vi "PrintDebugInfo.vi"(8 "error in (no error)":errorcluster, 11 "CLabVIEWContainer in":refnum<class "CLabVIEWContainer.lvclass">) -> (0 "error out":errorcluster, 1 "Debug string":string, 3 "CLabVIEWContainer out":refnum<class "CLabVIEWContainer.lvclass">)   [LabVIEW 2020, in "LabVIEWContainers.lvlib" / "CLabVIEWContainer.lvclass"]
uses:
  CLabVIEWContainer.lvclass
  CLabVIEWContainer.lvclass/CLabVIEWContainer.ctl
  obj/Addons/LabVIEWItem.lvlibp/LabVIEWItem/CLabVIEWItem/CLabVIEWItem.lvclass
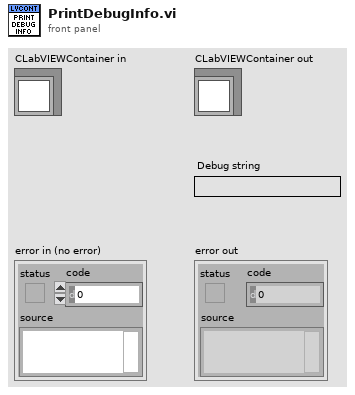
[diagram p1: front panel]
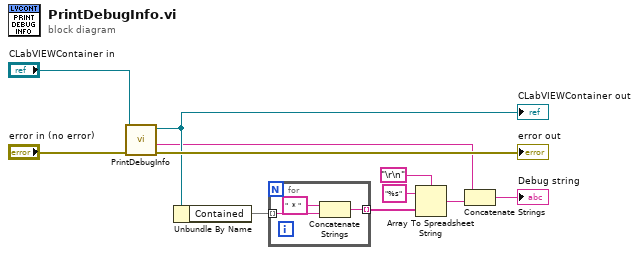
[diagram p0: block diagram]
diagram:
  n1 = call-parent "PrintDebugInfo.vi"("error in (no error)"="error in (no error)", "CLabVIEWItem in"="CLabVIEWContainer in") -> ("error out"=→"error out":errorcluster, "Debug string"=w2:string, "CLabVIEWItem out"=w8:refnum<class "CLabVIEWContainer.lvclass">)  [unwired: 7 in]
  "CLabVIEWContainer out" <- w8
  n2 = Unbundle By Name(w8) -> ("Contained"=w3:set{string})
  n3 = for {
    tunnel: w3 -> [w12] mode=indexing
    tunnel: [w14] -> w6 mode=indexing
    n4 = Concatenate Strings("  * " ("string"), w12) -> (w14:string)
  }
  n5 = Array To Spreadsheet String(delimiter (Tab)="\r\n", array=w6, 3:"%s" ("format string")) -> (spreadsheet string=w4:string)
  n6 = Concatenate Strings(w2, w4) -> (→"Debug string":string)
